vi "Start.vi"(8 "error in (no error)":errorcluster, 11 "service in":refnum<class "IcmMessageService.lvclass">) -> (0 "error out":errorcluster, 3 "service out":refnum<class "IcmMessageService.lvclass">)   [LabVIEW 2017, in "IcmMessageService.lvclass"]
doc: "Starts an NI InsightCM Server message bus session."
uses:
  <vilib>/addons/InsightCM/MessageBus/MessageService/IcmMessageService.lvclass
  <vilib>/addons/InsightCM/MessageBus/MessageService/IcmMessageService.lvclass/IcmMessageService.ctl
  C:/Program Files (x86)/National Instruments/LabVIEW 2017/vi.lib/addons/InsightCM/Binaries/LabviewMessageAdapter.dll
  Binaries/LabviewMessageAdapter.dll
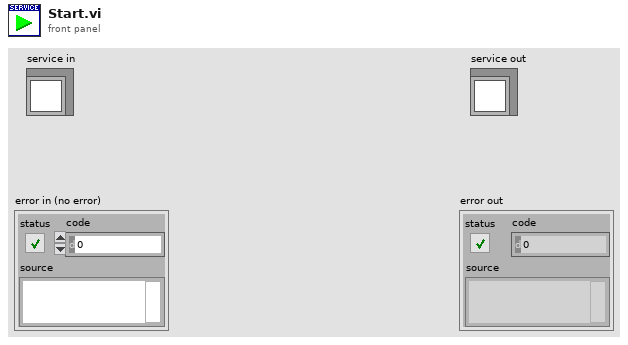
[diagram p1: front panel]
types:
  T1 = typedef "MessageServiceDvr.ctl" = refnum<data-value>
  T2 = typedef "MessageServiceData.ctl" = cluster{"Service":refnum<k24>}
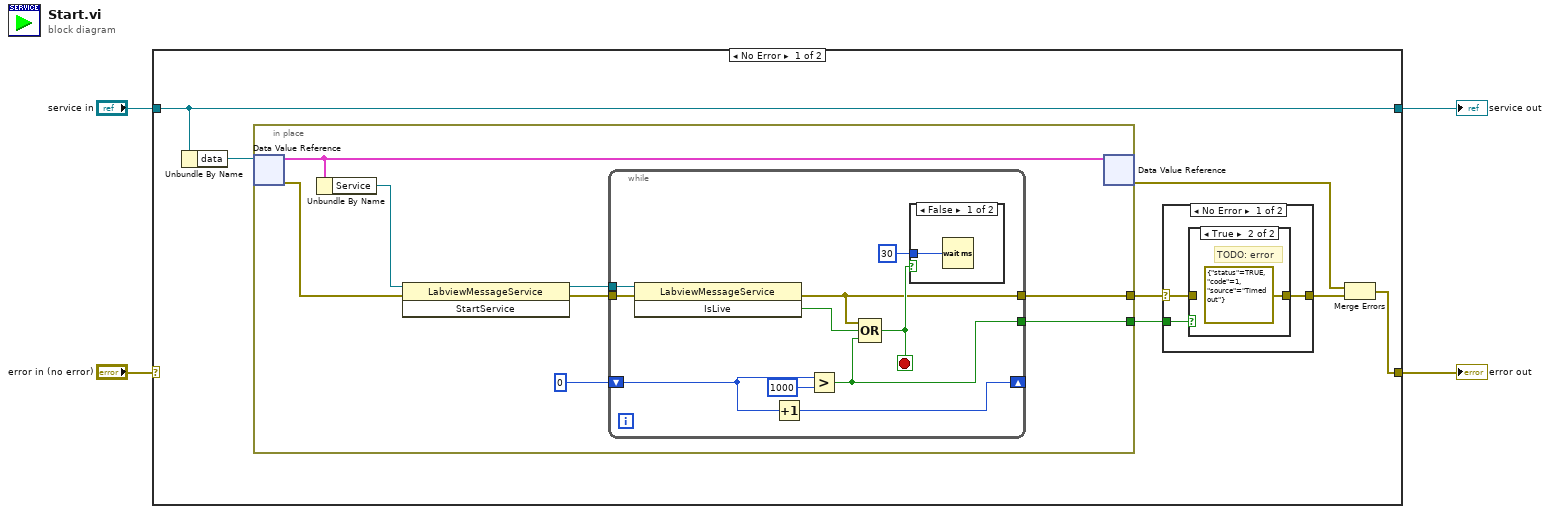
[diagram p0: block diagram]
diagram:
  n1 = case shown="No Error" "error in (no error)" {
    selector: "error in (no error)" -> [_ w38]
    tunnel: [w8 w38] -> w4
    tunnel: [w11 w37] -> w2
    tunnel: "service in" -> [w11 w37]
    frame No Error {
      n2 = Unbundle By Name(w11) -> ("data"=w10:T1)
      n3 = in-place {
        in-place-border: [w19] -> w7
        in-place-border: [w18] -> w6
        n4 = in-place-dvr #1(w10) -> (w25:T2, w23:errorcluster)
        n5 = Unbundle By Name(w25) -> ("Service"=w24:refnum<k24>)
        n6 = invoke class="LabviewMessageService" method="StartService"(reference=w24, error in=w23) -> (reference out=w20:refnum<k24>, error out=w21:errorcluster)  [unwired: 1 in, 1 out]
        n7 = while {
          tunnel: w20 -> [w29]
          tunnel: w21 -> [w28]
          tunnel: [w26] -> w19
          shift-right: [w31] -> _
          shift-left: 0 -> [w32]
          tunnel: [w30] -> w18
          stop <- w35 stop-if-true
          n8 = invoke class="LabviewMessageService" method="IsLive"(reference=w29, error in=w28) -> (error out=w26:errorcluster, "IsLive"=w27:bool)  [unwired: 1 in, 1 out]
          n9 = Increment(x=w32) -> (x+1=w31:i32)
          n10 = Greater?(x=w32, y=1000) -> (0:w30:bool)
          n11 = Compound Arithmetic op=OR(w26, w27, w30) -> (w35:bool)
          n12 = case shown="False" w35 {
            tunnel: u32 30 ("milliseconds to wait") -> [w36 _]
            frame False {
              n13 = Wait (ms)(milliseconds to wait=w36) -> ()  [unwired: 1 out]
            }
            frame True {
            }
          }
        }
        n14 = in-place-dvr #1(w25) -> (w9:errorcluster)  [unwired: 1 out]
      }
      n15 = case shown="No Error" w7 {
        selector: w7 -> [w12 w17]
        tunnel: [w13 w17] -> w5
        tunnel: w6 -> [w14 _]
        frame No Error {
          n16 = case shown="True" w14 {
            tunnel: [w15 errorcluster {"status"=TRUE, "code"=1, "source"="Timed out"} ("error IO")] -> w13
            tunnel: w12 -> [w15 _]
            frame False {
            }
            frame True {
              # "TODO: error"
            }
          }
        }
        frame Error {
        }
      }
      n17 = Merge Errors(w9, w5) -> (w8:errorcluster)
    }
    frame Error {
    }
  }
  "error out" <- w4
  "service out" <- w2
